vi "Taiko_Init.vi"(8 "error in (no error)":errorcluster, 9 "LBLHFeaturesRef":refnum<vi>, 10 "LBSysStatRef":refnum<vi>, 11 "Data":T1 {"TaggedValueList"."Tag" format="%x" items=["NONE"=0, "Locked"=16, "SoftLock"=17, "KeyLock"=18, "Class_IV_Lock"=20, "Interlock"=24, "LaserMode"=32, "LDH_PulsePowerTable"=33, "TriggerMode"=48, "TriggerLevelRaw"=64, "TriggerLevelRawLoLimit"=65, "TriggerLevelRawHiLimit"=66, "TriggerLevel"=72, "TriggerLevelLoLimit"=73, "TriggerLevelHiLimit"=74, "FastGate"=80, "FastGateImp"=96, "SlowGate"=112, "TargetTempRaw"=144, "TargetTempRawLoLimit"=145, "TargetTempRawHiLimit"=146, "CurrentTempRaw"=148, "CaseTempRaw"=149, "TargetTemp"=152, "TargetTempLoLimit"=153, "TargetTempHiLimit"=154, "CurrentTemp"=156, "CaseTemp"=157, "TempScale"=159, "Frequency"=168, "FrequencyLoLimit"=169, "FrequencyHiLimit"=170, "PulsePowerRaw"=176, "PulsePowerRawLoLimit"=177, "PulsePowerRawHiLimit"=178, "PulsePowerPermille"=180, "PulseShape"=181, "PulsePower"=184, "PulsePowerLoLimit"=185, "PulsePowerHiLimit"=186, "PulsePowerNanowatt"=188, "PulsePowerVoltage"=190, "PulseEnergy"=191, "CwPowerRaw"=192, "CwPowerRawLoLimit"=193, "CwPowerRawHiLimit"=194, "CwPowerPermille"=196, "CwPower"=200, "CwPowerLoLimit"=201, "CwPowerHiLimit"=202, "CwPowerMicroWatt"=204, "BurstLen"=208, "BurstPeriod"=224, "LDH_Fan"=240, "UI_Exclusive"=256]}) -> (0 "error out":errorcluster, 1 "Status":string, 2 "LHInfoData":string[][](array[string]), 3 "Data out":T1 {"TaggedValueList"."Tag" format="%x" items=["NONE"=0, "Locked"=16, "SoftLock"=17, "KeyLock"=18, "Class_IV_Lock"=20, "Interlock"=24, "LaserMode"=32, "LDH_PulsePowerTable"=33, "TriggerMode"=48, "TriggerLevelRaw"=64, "TriggerLevelRawLoLimit"=65, "TriggerLevelRawHiLimit"=66, "TriggerLevel"=72, "TriggerLevelLoLimit"=73, "TriggerLevelHiLimit"=74, "FastGate"=80, "FastGateImp"=96, "SlowGate"=112, "TargetTempRaw"=144, "TargetTempRawLoLimit"=145, "TargetTempRawHiLimit"=146, "CurrentTempRaw"=148, "CaseTempRaw"=149, "TargetTemp"=152, "TargetTempLoLimit"=153, "TargetTempHiLimit"=154, "CurrentTemp"=156, "CaseTemp"=157, "TempScale"=159, "Frequency"=168, "FrequencyLoLimit"=169, "FrequencyHiLimit"=170, "PulsePowerRaw"=176, "PulsePowerRawLoLimit"=177, "PulsePowerRawHiLimit"=178, "PulsePowerPermille"=180, "PulseShape"=181, "PulsePower"=184, "PulsePowerLoLimit"=185, "PulsePowerHiLimit"=186, "PulsePowerNanowatt"=188, "PulsePowerVoltage"=190, "PulseEnergy"=191, "CwPowerRaw"=192, "CwPowerRawLoLimit"=193, "CwPowerRawHiLimit"=194, "CwPowerPermille"=196, "CwPower"=200, "CwPowerLoLimit"=201, "CwPowerHiLimit"=202, "CwPowerMicroWatt"=204, "BurstLen"=208, "BurstPeriod"=224, "LDH_Fan"=240, "UI_Exclusive"=256]}, 4 "Features":string)   [LabVIEW 2010]
uses:
  _lib/PDLM/pdlm_lib_x86_x64_UIThread.llb/PDLM_NamedBit.ctl
  _lib/PDLM/pdlm_lib_x86_x64_UIThread.llb/PDLM_Tag.ctl
  _lib/PDLM/pdlm_lib_x86_x64_UIThread.llb/PDLM_TaggedValue.ctl
  _lib/PDLM/pdlm_lib_x86_x64_UIThread.llb/PDLM_LHFeatures.ctl
  _lib/PDLM/pdlm_lib_x86_x64_UIThread.llb/PDLM_TaggedValueList.ctl
  Types/Taiko_Data.ctl
  Types/ControlAttributes.ctl
  Types/ScaleDisplayParams.ctl
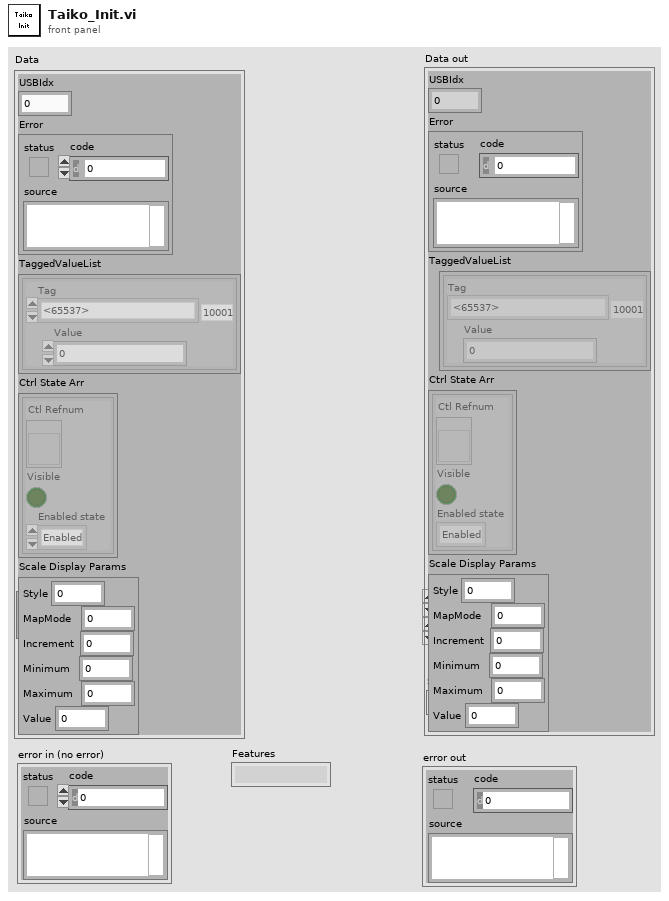
[diagram p1: front panel]
types:
  T1 = typedef "Taiko_Data.ctl" = cluster{"USBIdx":i32, "Error":errorcluster, "TaggedValueList":T2, "Ctrl State Arr":T5[], "Scale Display Params":T6}
  T2 = typedef "PDLM_TaggedValueList.ctl" = T3[]
  T3 = typedef "PDLM_TaggedValue.ctl" = cluster{"Tag":T4, "Value":u32}
  T4 = typedef "PDLM_Tag.ctl" = u32
  T5 = typedef "ControlAttributes.ctl" = cluster{"Ctl Refnum":refnum<vi>, "Visible":bool, "Enabled state":enum8{"Enabled", "Disabled", "Disabled and Grayed Out"}}
  T6 = typedef "ScaleDisplayParams.ctl" = cluster{"Style":u8, "MapMode":u8, "Increment":dbl, "Minimum":dbl, "Maximum":dbl, "Value":dbl}
  T7 = typedef "PDLM_LHFeatures.ctl" = T8[]
  T8 = typedef "PDLM_NamedBit.ctl" = cluster{"StatName":string, "StatBit":bool}
  T9 = typedef "LVStringsAndValuesArrayTypeDef_U32.ctl" = cluster{"String":string, "Value":u32}[]
  T10 = typedef "PDLM_LHInfo.ctl" = cluster{"LType":string, "Date":string, "LClass":string}
  T11 = typedef "PDLM_LHData.ctl" = cluster{"SerNo":u32, "Features":u32, "FreqMin":u32, "FreqMax":u32, "CwPowerMax":u32, "PulsePowerMax":u32, "WavelengthNominal":u16, "CaseTempMax":u16, "Protection":bool, "LHTypeCtrlVoltage":u16, "LHMaxVoltage":u16, "CurrentTEP12V":u16, "LaserType":T12, "LHVersion":T13, "CalWarrentHours":u16}
  T12 = typedef "PDLM_LHData_LaserType.ctl" = u16
  T13 = typedef "PDLM_LHVersion.ctl" = cluster{"Major":u16, "Minor":u16}
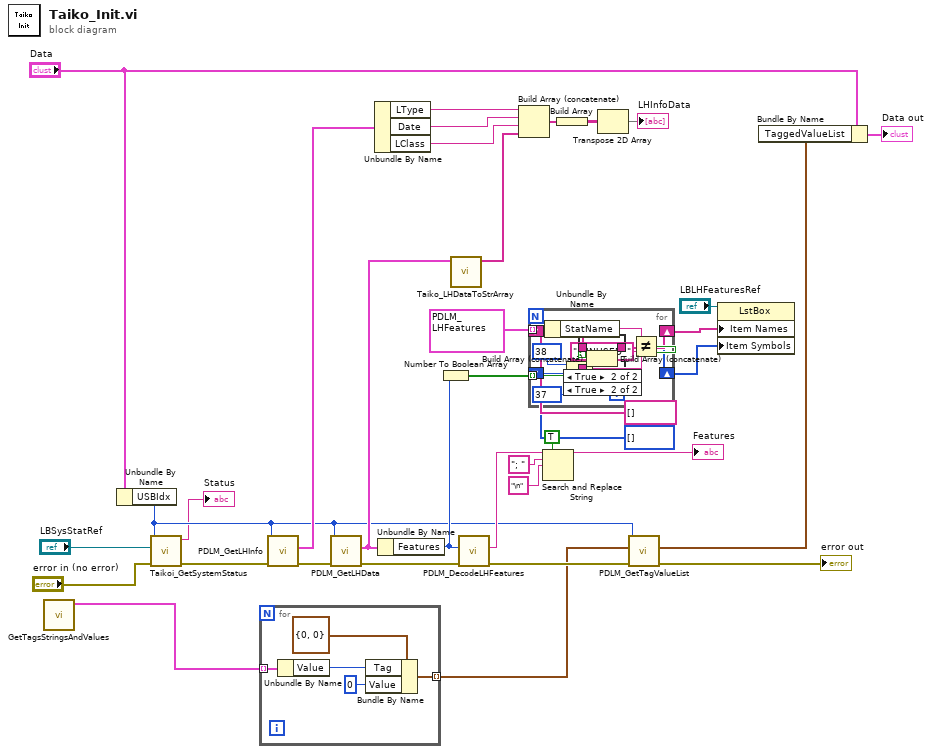
[diagram p0: block diagram]
diagram:
  n1 = call "GetTagsStringsAndValues.vi"() -> ("Strings And Values []"=w3:T9)  [unwired: 11 in]
  n2 = Unbundle By Name("Data") -> ("USBIdx"=w8:i32)
  n3 = call "Taikoi_GetSystemStatus.vi"("error in (no error)"="error in (no error)", "LBSysStatRef"="LBSysStatRef", "USBIdx"=w8) -> ("error out"=w9:errorcluster, "Status"=→"Status":string)  [unwired: 5 in, 2 out]
  n4 = for {
    tunnel: w3 -> [w41] mode=indexing
    tunnel: [w37] -> w13 mode=indexing
    n5 = Unbundle By Name(w41) -> ("Value"=w39:u32)
    n6 = Bundle By Name(cluster=T3 {"Tag"=0, "Value"=0} ("TaggedValue"), "Tag"=w39, "Value"=u32 0) -> (w37:T3)
  }
  n7 = call "PDLM_GetLHInfo.vi"("error in (no error)"=w9, "USBIdx"=w8) -> ("error out"=w36:errorcluster, "LHInfo"=w31:T10)  [unwired: 7 in, 1 out]
  n8 = call "PDLM_GetLHData.vi"("error in (no error)"=w36, "USBIdx"=w8) -> ("error out"=w29:errorcluster, "Data"=w30:T11)  [unwired: 7 in, 1 out]
  n9 = Unbundle By Name(w31) -> ("LType"=w6:string, "Date"=w5:string, "LClass"=w4:string)
  n10 = Unbundle By Name(w30) -> ("Features"=w25:u32)
  n11 = Number To Boolean Array(number=w25) -> (Boolean array=w26:bool[])
  n12 = call "Taiko_LHDataToStrArray.vi"("LHData"=w30) -> ("StrArray"=w34:string[])  [unwired: 10 in]
  n13 = call "PDLM_DecodeLHFeatures.vi"("error in (no error)"=w29, "features"=w25) -> ("error out"=w28:errorcluster, "Buffer"=w17:string)  [unwired: 7 in, 1 out]
  n14 = Build Array (concatenate)(w6, w5, w4, w34) -> (w32:string[])
  n15 = for {
    tunnel: w26 -> [w52] mode=indexing
    tunnel: T7 [{"StatName"="CW_CAPABILITY", "StatBit"=FALSE}, {"StatName"="_UNUSED_", "StatBit"=FALSE}, {"StatName"="_UNUSED_", "StatBit"=FALSE}, {"StatName"="_UNUSED_", "StatBit"=FALSE}, {"StatName"="BURST_CAPABILITY", "StatBit"=FALSE}, {"StatName"="_UNUSED_", "StatBit"=FALSE}, {"StatName"="EXTERNAL_TRIGGERABLE_BURSTS", "StatBit"=FALSE}, {"StatName"="EXTERNAL_TRIGGERABLE_PULSES", "StatBit"=FALSE}, {"StatName"="WL_TUNABLE", "StatBit"=FALSE}, {"StatName"="_UNUSED_", "StatBit"=FALSE}, {"StatName"="_UNUSED_", "StatBit"=FALSE}, {"StatName"="_UNUSED_", "StatBit"=FALSE}, {"StatName"="_UNUSED_", "StatBit"=FALSE}, {"StatName"="_UNUSED_", "StatBit"=FALSE}, {"StatName"="_UNUSED_", "StatBit"=FALSE}, {"StatName"="_UNUSED_", "StatBit"=FALSE}, {"StatName"="COOLING_FAN", "StatBit"=FALSE}, {"StatName"="SWITCHABLE_FAN", "StatBit"=FALSE}, {"StatName"="_UNUSED_", "StatBit"=FALSE}, {"StatName"="_UNUSED_", "StatBit"=FALSE}, {"StatName"="_UNUSED_", "StatBit"=FALSE}, {"StatName"="_UNUSED_", "StatBit"=FALSE}, {"StatName"="_UNUSED_", "StatBit"=FALSE}, {"StatName"="_UNUSED_", "StatBit"=FALSE}, {"StatName"="_UNUSED_", "StatBit"=FALSE}, {"StatName"="_UNUSED_", "StatBit"=FALSE}, {"StatName"="_UNUSED_", "StatBit"=FALSE}, {"StatName"="_UNUSED_", "StatBit"=FALSE}, {"StatName"="_UNUSED_", "StatBit"=FALSE}, {"StatName"="_UNUSED_", "StatBit"=FALSE}, {"StatName"="_UNUSED_", "StatBit"=FALSE}, {"StatName"="_UNUSED_", "StatBit"=FALSE}] ("LHFeatures") -> [w53] mode=indexing
    shift-right: [w44] -> w23
    shift-left: string[] [] ("Array") -> [w45]
    shift-right: [w42] -> w22
    shift-left: i32[] [] ("Array") -> [w43]
    n16 = Unbundle By Name(w53) -> ("StatName"=w48:string)
    n17 = Select(t=38, s=w52, f=37) -> (s? t:f=w49:i32)
    n18 = Not Equal?(x=w48, y="_UNUSED_") -> (x != y?=w46:bool)
    n19 = case shown="True" w46 {
      tunnel: w43 -> [w54 w56]
      tunnel: w49 -> [_ w55]
      tunnel: [w54 w57] -> w42
      frame False {
      }
      frame True {
        n20 = Build Array (concatenate)(w56, w55) -> (w57:i32[])
      }
    }
    n21 = case shown="True" w46 {
      tunnel: w45 -> [w58 w60]
      tunnel: w48 -> [_ w59]
      tunnel: [w58 w61] -> w44
      frame False {
      }
      frame True {
        n22 = Build Array (concatenate)(w60, w59) -> (w61:string[])
      }
    }
  }
  n23 = Search and Replace String(replace all?=TRUE ("replace all? (F)"), input string=w17, search string="; ", replace string="\n" ("replace string (\"\")")) -> (result string=→"Features":string)  [unwired: 4 in, 3 out]
  n24 = Build Array(w32) -> (w33:string[][])
  n25 = Transpose 2D Array(2D array=w33) -> (transposed array=→"LHInfoData":string[][])
  n26 = call "PDLM_GetTagValueList.vi"("error in (no error)"=w28, "TaggedValueList"=w13, "USBIdx"=w8) -> ("error out"=→"error out":errorcluster, "TaggedValueList out"=w14:T2)  [unwired: 6 in, 1 out]
  n27 = property class="LstBox"(reference="LBLHFeaturesRef", "Item Names"=w23, "Item Symbols"=w22) -> ()  [unwired: 1 in, 2 out]
  n28 = Bundle By Name(cluster="Data", "TaggedValueList"=w14) -> (→"Data out":T1)
